vi "PF2PS.vi"(8 "error in":errorcluster, 9 "Setpoint":dbl, 10 "Run":bool, 11 "PS in":refnum<class "Power Supply.lvclass">) -> (0 "error out":errorcluster, 3 "PS out":refnum<class "Power Supply.lvclass">)   [LabVIEW 2019, in "Power Supply.lvlib" / "Power Supply.lvclass"]
uses:
  Power Supply.lvclass
  Power Supply.lvclass/Power Supply.ctl
  <userlib>/_MGI/Application Control/MGI Gray if/MGI Gray if False.vi
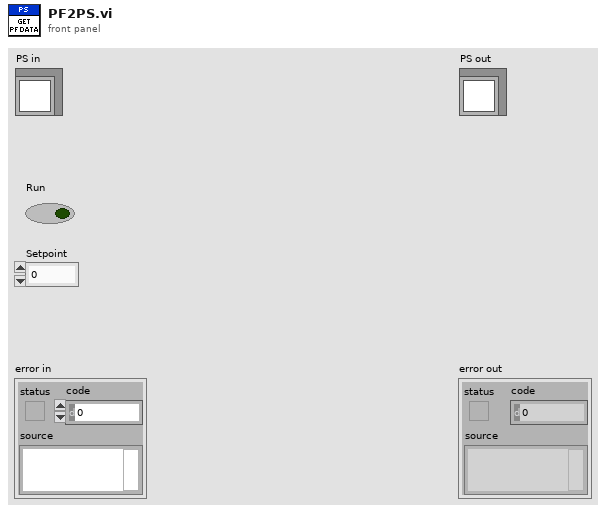
[diagram p1: front panel]
types:
  T1 = enum8{"Enabled", "Disabled", "Disabled and Grayed Out"}
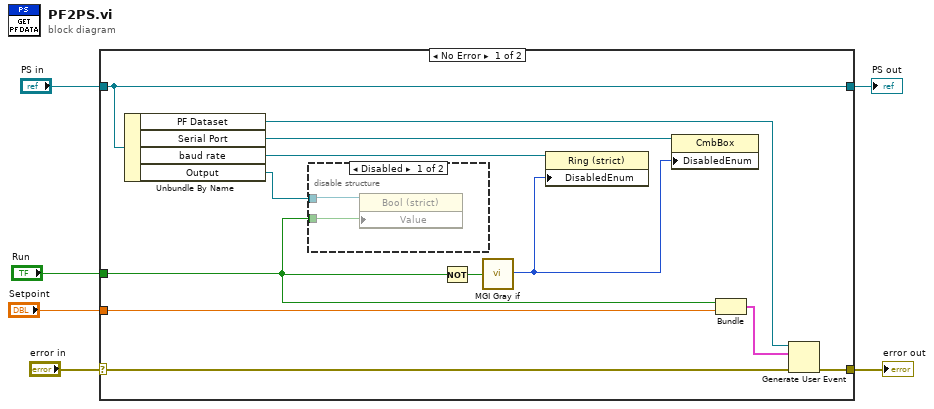
[diagram p0: block diagram]
diagram:
  n1 = case shown="No Error" "error in" {
    selector: "error in" -> [w16 w22]
    tunnel: [w13 w22] -> w6
    tunnel: [w12 w21] -> w5
    tunnel: "PS in" -> [w12 w21]
    tunnel: "Setpoint" -> [w11 _]
    tunnel: "Run" -> [w7 _]
    frame No Error {
      n2 = Unbundle By Name(w12) -> ("PF Dataset"=w18:refnum<user-event>, "Serial Port"=w15:refnum<vi>, "baud rate"=w14:refnum<vi>, "Output"=w8:refnum<vi>)
      n3 = disable-structure shown="Disabled" {
        disable-tunnel: w8 -> [w20 _]
        disable-tunnel: w7 -> [w19 _]
        frame Disabled {
          n4 = property class="Bool (strict)"(reference=w20, "Value"=w19) -> ()  [unwired: 1 in, 2 out]
        }
        frame Enabled {
        }
      }
      n5 = Not(x=w7) -> (.not. x?=w9:bool)
      n6 = call-poly <userlib>:"MGI Gray if.vi"("Boolean"=w9) -> ("Disabled"=w10:T1)
      n7 = property class="Ring (strict)"(reference=w14, "DisabledEnum"=w10) -> ()  [unwired: 1 in, 2 out]
      n8 = property class="CmbBox"(reference=w15, "DisabledEnum"=w10) -> ()  [unwired: 1 in, 2 out]
      n9 = Bundle("Run"=w7, "Setpoint"=w11) -> (w17:cluster{"Run":bool, "Setpoint":dbl})  [unwired: 1 in]
      n10 = Generate User Event(user event=w18, event data cluster=w17, error in=w16) -> (error out=w13:errorcluster)  [unwired: 1 in, 1 out]
    }
    frame Error {
    }
  }
  "error out" <- w6
  "PS out" <- w5
